vi "PiezoWaveGeneration.vi"(3 "WAVE":T1={"Speed"=0.0, "Stiffness (0.95)"=0.95, "Linear Stroke"=0.0, "Delay"=0.0} {"Delay" format="%.2f"; "Linear Stroke" format="%.2f"; "Stiffness (0.95)" format="%.2f"; "Speed" format="%.2f"}, 9 "error in (no error)":errorcluster) -> (0 "Graphe":waveform(dbl)(graph), 6 "error out":errorcluster)   [LabVIEW 2009]
uses:
  Controls/PIEZO.WAVE.ctl
  <vilib>/Waveform/WDTOps.llb/WDT Append Waveforms DBL.vi
  <vilib>/Waveform/WDTOps.llb/WDT Number of Waveform Samples DBL.vi
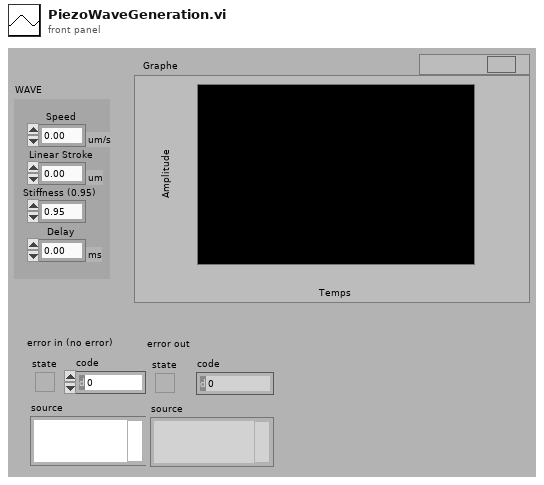
[diagram p1: front panel]
types:
  T1 = typedef "PIEZO.WAVE.ctl" = cluster{"Speed":dbl[unit], "Stiffness (0.95)":dbl, "Linear Stroke":dbl[unit], "Delay":dbl[unit]}
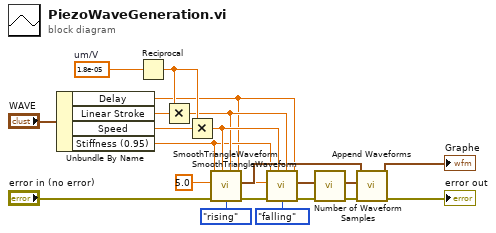
[diagram p0: block diagram]
diagram:
  w1 = dbl[unit] 5.0 ("Offset")
  w17 = dbl[unit] 1.8e-05  # um/V
  n1 = Unbundle By Name("WAVE") -> ("Delay"=w5:dbl[unit], "Linear Stroke"=w6:dbl[unit], "Speed"=w7:dbl[unit], "Stiffness (0.95)"=w8:dbl)
  n2 = Reciprocal(x=w17) -> (1/x=w15:dbl[unit])
  n3 = Multiply(x=w15, y=w6) -> (x*y=w14:dbl[unit])
  n4 = Multiply(x=w15, y=w7) -> (x*y=w16:dbl[unit])
  n5 = call "SmoothTriangleWaveform.vi"("error in"="error in (no error)", "Direction"=enum16{"rising", "falling"}."rising", "Offset"=w1, "Stiffness"=w8, "Speed"=w16, "Linear Amplitude"=w14, "Delay"=w5) -> ("error out"=w18:errorcluster, "Smooth Triangle Waveform"=w13:waveform(dbl))  [unwired: 2 in]
  n6 = call "SmoothTriangleWaveform.vi"("error in"=w18, "Direction"=enum16{"rising", "falling"}."falling", "Offset"=w1, "Stiffness"=w8, "Speed"=w16, "Linear Amplitude"=w14, "Delay"=w5) -> ("error out"=w12:errorcluster, "Smooth Triangle Waveform"=w10:waveform(dbl))  [unwired: 2 in]
  n7 = call-poly <vilib>:"Number of Waveform Samples.vi"("error in (no error)"=w12, "waveform in"=w10) -> ("error out"=w11:errorcluster, "waveform out"=w9:waveform(dbl))  [unwired: 7 in, 1 out]
  n8 = call-poly <vilib>:"Append Waveforms.vi"("error in (no error)"=w11, "waveform B"=w9, "waveform A"=w13) -> ("error out"=→"error out":errorcluster, "waveform out"=→"Graphe":waveform(dbl))  [unwired: 7 in]
